vi "Get Outgoing Signal Names.vi"(8 "error in (no error)":errorcluster, 11 "Port in":T1 format="%.0x") -> (0 "error out":errorcluster, 1 "signal names":string[](array[string]), 2 "signals":T1[](array[typedef]) format="%.0x", 3 "Port out":T1 format="%.0x")   [LabVIEW 2020, in "Communication Bus Template Engine.lvlib" / "Implementation.lvlib" / "Execution Unit Factory.lvclass"]
uses:
  Execution Unit Factory.lvclass
  Scripting/Communication Bus Template Scripting.lvlib
  <vilib>/NI VeriStand/Custom Device API/Custom Device API.lvlib
  <vilib>/NI VeriStand/Custom Device API/Custom Device Item Ref.ctl
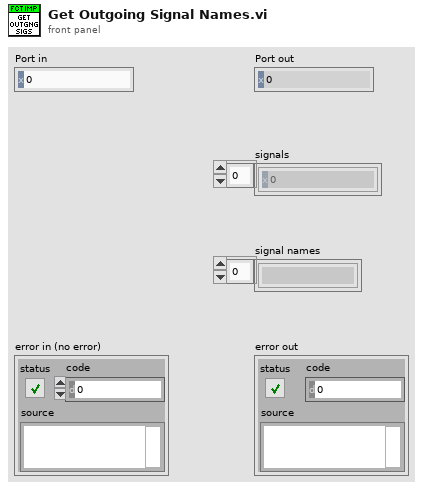
[diagram p1: front panel]
types:
  T1 = typedef "Custom Device API.lvlib/Custom Device Item Ref.ctl" = u64
  T2 = typedef "Custom Device API.lvlib/Custom Device Item Info.ctl" = cluster{"Name":string, "Is Channel":bool, "GUID":string, "Is Waveform":bool}
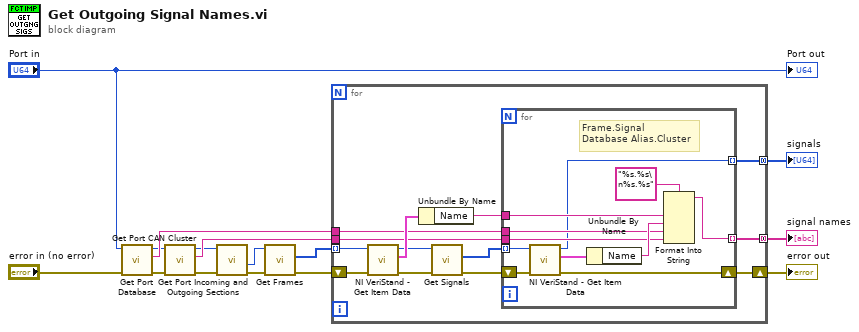
[diagram p0: block diagram]
diagram:
  n1 = call "Get Port Database.vi"("error in"="error in (no error)", "Port Ref"="Port in") -> ("error out"=w10:errorcluster, "Database Name"=w13:string, "Port Ref out"=w9:T1)  [unwired: 5 in, 2 out]
  n2 = call "Get Port CAN Cluster.vi"("error in"=w10, "Port Ref"=w9) -> ("error out"=w3:errorcluster, "CAN Cluster"=w14:string, "Port Ref out"=w4:T1)  [unwired: 7 in]
  n3 = call "Get Port Incoming and Outgoing Sections.vi"("error in"=w3, "Port Ref"=w4) -> ("error out"=w2:errorcluster, "Outgoing"=w1:T1)  [unwired: 6 in, 2 out]
  n4 = call "Get Frames.vi"("error in"=w2, "Incoming/Outgoing in"=w1) -> ("error out"=w12:errorcluster, "Frames"=w11:T1[])  [unwired: 7 in, 1 out]
  n5 = for {
    tunnel: w11 -> [w27] mode=indexing
    shift-right: [w25] -> w7
    shift-left: w12 -> [w26]
    tunnel: w13 -> [w16]
    tunnel: w14 -> [w23]
    tunnel: [w22] -> w6 mode=concatenating
    tunnel: [w21] -> w5 mode=concatenating
    n6 = call <vilib>:"NI VeriStand - Get Item Data.vi"("error in (no error)"=w26, "Item Ref in"=w27) -> ("error out"=w19:errorcluster, "Item Info"=w28:T2, "Item Ref out"=w20:T1)  [unwired: 6 in, 1 out]
    n7 = Unbundle By Name(w28) -> ("Name"=w24:string)
    n8 = call "Get Signals.vi"("error in"=w19, "Frame in"=w20) -> ("error out"=w18:errorcluster, "Signals"=w17:T1[])  [unwired: 7 in, 1 out]
    n9 = for {
      shift-right: [w36] -> w25
      shift-left: w18 -> [w37]
      tunnel: w17 -> [w31] mode=indexing
      tunnel: w24 -> [w38]
      tunnel: w16 -> [w33]
      tunnel: w23 -> [w32]
      tunnel: [w30] -> w22 mode=indexing
      tunnel: [w29] -> w21 mode=indexing
      # "Frame.Signal\nDatabase Alias.Cluster"
      n10 = call <vilib>:"NI VeriStand - Get Item Data.vi"("error in (no error)"=w37, "Item Ref in"=w31) -> ("error out"=w36:errorcluster, "Item Info"=w35:T2, "Item Ref out"=w29:T1)  [unwired: 6 in, 1 out]
      n11 = Unbundle By Name(w35) -> ("Name"=w34:string)
      n12 = Format Into String(format string="%s.%s\n%s.%s", w38, w34, w33, w32) -> (resulting string=w30:string)  [unwired: 2 in, 1 out]
    }
  }
  "error out" <- w7
  "signal names" <- w6
  "signals" <- w5
  "Port out" <- "Port in"
